vi "Merge Data.vi"(8 "error in (no error)":errorcluster, 10 "From":refnum<class "Server Message.lvclass">, 11 "Typed Response in":refnum<class "Response.lvclass">) -> (0 "error out":errorcluster, 3 "Typed Response out":refnum<class "Response.lvclass">)   [LabVIEW 2022 SP3, in "obs-websocket-lv.lvlib" / "Response.lvclass"]
uses:
  Response.lvclass
  Response.lvclass/Response.ctl
  Server Message/Server Message.lvclass
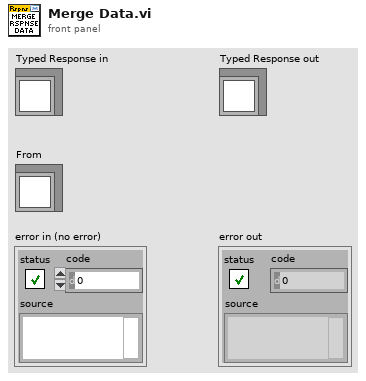
[diagram p1: front panel]
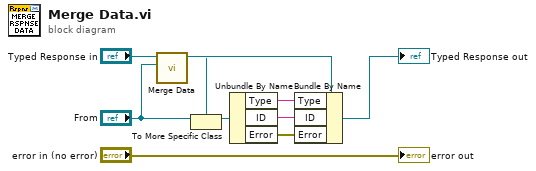
[diagram p0: block diagram]
diagram:
  n1 = call-parent "Merge Data.vi"("From"="From", "Server Message in"="Typed Response in") -> ("Server Message out"=w4:refnum<class "Response.lvclass">)  [unwired: 8 in, 1 out]
  n2 = To More Specific Class(target class="Typed Response in", reference="From") -> (specific class reference=w1:refnum<class "Response.lvclass">)  [unwired: 1 in, 1 out]
  n3 = Unbundle By Name(w1) -> ("Type"=w8:string, "ID"=w7:string, "Error"=w6:errorcluster)
  n4 = Bundle By Name(cluster=w4, "Type"=w8, "ID"=w7, "Error"=w6) -> (→"Typed Response out":refnum<class "Response.lvclass">)
  "error out" <- "error in (no error)"
